vi "Configure ESR query.vi"(8 "error in (no error)":errorcluster, 11 "VISA resource name":refnum<visa-resource-name>) -> (0 "error out":errorcluster, 2 "Result":string, 3 "VISA resource name out":refnum<visa-resource-name>)   [LabVIEW 2025]
panel:
  # "*ESR?"
  # "Standar Event Status Register query"
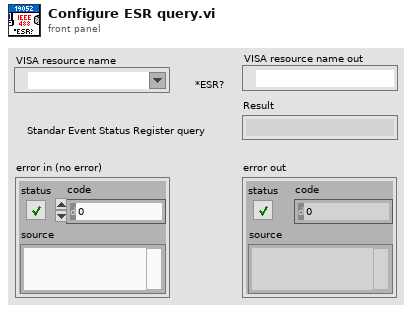
[diagram p1: front panel]
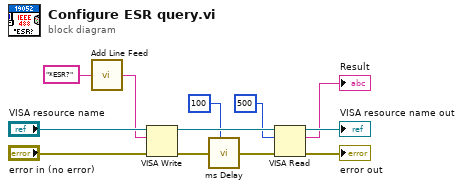
[diagram p0: block diagram]
diagram:
  n1 = call <instrlib>:"Add Line Feed.vi"("Command string"="*ESR?") -> ("Concatenated string"=w1:string)  [unwired: 4 in]
  n2 = VISA Write(VISA resource name="VISA resource name", write buffer=w1, error in (no error)="error in (no error)") -> (VISA resource name out=w5:refnum<visa-resource-name>, error out=w7:errorcluster)  [unwired: 1 out]
  n3 = call <instrlib>:"ms Delay.vi"("miliseconds to wait"=u32 100 ("Time Delay S"), "error in (no error)"=w7) -> ("error out"=w6:errorcluster)  [unwired: 6 in, 1 out]
  n4 = VISA Read(VISA resource name=w5, byte count=u32 500 ("byte count (0)"), error in (no error)=w6) -> (VISA resource name out=→"VISA resource name out":refnum<visa-resource-name>, read buffer=→"Result":string, error out=→"error out":errorcluster)  [unwired: 1 out]
